vi "Transcript VIs.vi"() -> ()   [LabVIEW 2014]
panel:
  out "transcripted code":string="#include <StandardCplusplus.h>\r\n#include <vector>\r\n#include <ArduinoBasicFunctions.h>\r\n#include <CircularBuffer.h>\nusing namespace std;\r\nCircularBuffer<String,1> shiftRegister_438;\r\nbool shiftRegisterInitBool_438 = true;\r\n\r\nCircularBuffer<double,1> shiftRegister_460;\r\nbool shiftRegisterInitBool_460 = true;\r\n\r\n\nString Example_Shift_Register_Loop_1(String userString1,double numberA){\n    double wireUID_1011_;\r\n    String wireUID_1506_;\r\n    double wireUID_1464_;\r\n    String wireUID_1031_;\r\n    /***** BEGIN WhileLoop ********/\n    CircularBuffer<double,1> shiftRegister_1173;\r\n    bool shiftRegisterInitBool_1173 = true;\r\n    \r\n    CircularBuffer<String,1> shiftRegister_1326;\r\n    bool shiftRegisterInitBool_1326 = true;\r\n    \r\n    bool wireUID_333_ = false; //LoopEndRef.\n    int iteratorUID_428 = 0; //loop iterator\n    do{\n        if (shiftRegisterInitBool_438){\n            shiftRegister_438.push(wireUID_1031_);\r\n            shiftRegisterInitBool_438 = false;\n        }\r\n        if (shiftRegisterInitBool_460){\n            shiftRegister_460.push(wireUID_1011_);\r\n            shiftRegisterInitBool_460 = false;\n        } //shift register init\n        double wireUID_499_ = shiftRegister_460.shift();\r\n        String wireUID_488_;\r\n        double wireUID_477_;\r\n        String wireUID_466_ = shiftRegister_438.shift();\r\n        /***** BEGIN WhileLoop ********/\n        bool wireUID_1433_ = false; //LoopEndRef.\n        int iteratorUID_989 = 0; //loop iterator\n        do{\n            if (shiftRegisterInitBool_1173){\n                shiftRegister_1173.push(wireUID_499_);\r\n                shiftRegisterInitBool_1173 = false;\n            }\r\n            if (shiftRegisterInitBool_1326){\n                shiftRegister_1326.push(wireUID_466_);\r\n                shiftRegisterInitBool_1326 = false;\n            } //shift register init\n            double wireUID_1192_;\r\n            String wireUID_1322_ = shiftRegister_1326.shift();\r\n            String wireUID_1295_;\r\n            double wireUID_1118_ = shiftRegister_1173.shift();\r\n            double wireUID_1150_ = 4.200000;\r\n            bool wireUID_1116_;\r\n            wireUID_1116_ = (wireUID_1150_ >= wireUID_1118_);\r\n            /***** BEGIN CaseStructure ********/\n            switch(wireUID_1116_){\n                case false:\n                {\n                    String wireUID_1401_ = \"Hello world.\";\r\n                    double wireUID_1266_ = 0.000000;\r\n                     /* C code */\n                    wireUID_1192_ = wireUID_1266_;\r\n                    wireUID_1295_ = wireUID_1401_; /* output assgn. */\n                }\n                break;\r\n                case true:\n                {\n                    String wireUID_1313_ = wireUID_1322_;\r\n                    double wireUID_1210_ = wireUID_1118_;\r\n                     /* C code */\n                    wireUID_1192_ = wireUID_1210_;\r\n                    wireUID_1295_ = wireUID_1313_; /* output assgn. */\n                }\n                break;\n            }\n            /****** END CaseStructure ********/\r\n             //C code\n            \r\n            shiftRegister_1173.push(wireUID_1192_);\r\n            shiftRegister_1326.push(wireUID_1295_); //output assgn.\n            iteratorUID_989++; //iterator increment\n        }while(!wireUID_1433_); //negation because in LabVIEW it is when stop (oposite)\n        /****** END WhileLoop */\r\n         //C code\n        \r\n        shiftRegister_438.push(wireUID_488_);\r\n        shiftRegister_460.push(wireUID_477_); //output assgn.\n        iteratorUID_428++; //iterator increment\n    }while(!wireUID_333_); //negation because in LabVIEW it is when stop (oposite)\n    /****** END WhileLoop */\r\n    \n}\n\nvoid setup(){}\nvoid loop(){\n    Example_Shift_Register_Loop_1();\n}\n"
  in  "vi path":path=path "C:/Users/miesizelezo/Documents/LabVIEW/LabVIEW-Universal-Transcriptor/Test/Examples For Parsing/Example FlatSequence 1.vi"
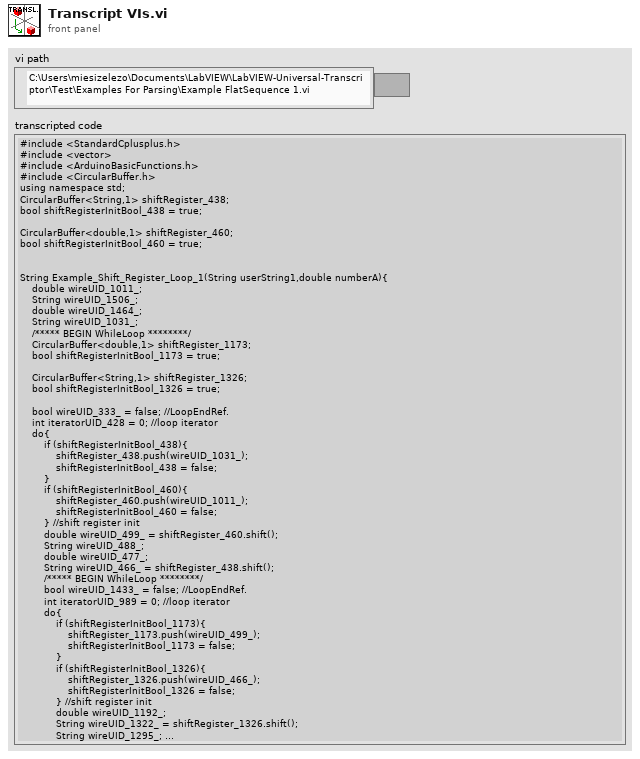
[diagram p1: front panel]
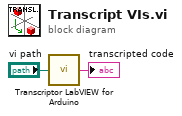
[diagram p0: block diagram]
diagram:
  n1 = call <vilib>:"Transcriptor LabVIEW for Arduino.vi"("vi path"="vi path") -> ("transcripted code"=→"transcripted code":string)
